vi "CyberSim.vi"() -> ()   [LabVIEW 2015]
doc: "Top-level VI to run one simulation of the iRobot and environment."
uses:
  CyberSim interface/Simulation Configuration.ctl
  autograder/feedbackMode.ctl
  shared/Kobuki Sensor Display.ctl
  <vilib>/Utility/miscctls.llb/LVRectTypeDef.ctl
  shared/Accelerometer.ctl
  <vilib>/Utility/miscctls.llb/LVPositionTypeDef.ctl
panel:
  out "size(s) 3":i32
  out "Display:Primary Workspace":T1
  out "Front Panel Window:Panel Bounds":T1
  in  "home camera":bool
  in  "stop":bool
  in  "start":bool
  in  "pause":bool
  in  "check grade":bool
  in  "exit":bool=TRUE
  out "Simulator Display":refnum<vi>(3d-picture)
  out "FullScreen":bool caption="--> Full Simulator Screens.\nPress \"ESC\" to exis full screen"
  in  "Change Sence":bool
  out "Sequence Number":i32
  out "Simulation Running":bool
  in  "Front Panel Tabs":T2(tab)=enum."Configuration"
  out "Statechart Diagram Display (supports LabVIEW Statecharts only)":picture
  out "Feedback":string
  in  "Simulation Configuration":T3={"maxTime"=inf, "enableVisualization"=TRUE, "Environment Definition"=path "Environment - Kobuki Hill Climb 1.xml", "Record Location"=path "Simulation Record.xml", "autograde?"=FALSE, "interactive?"=FALSE, "Feedback Mode"=enum."debug navigation", "Robot State Charts"=[path "../statechart/Simulation Statechart.vi"], "statechart"=path "../statechart/Simulation Statechart.vi"}
  in  "save configuration":bool
  in  "terminate at simulation end?":bool
  out "Simulation Time (s)":sgl=48.645 format="%7.3g"
  in  "play":bool
  out "?":T5={"Center Bump"=FALSE, "Left Wheel Drop"=FALSE, "Right Wheel Drop"=FALSE, "Left Bump"=FALSE, "Right Bump"=FALSE, "Left Cliff"=FALSE, "Center Cliff"=FALSE, "Right Cliff"=FALSE, "Net Dist (mm)"=3605, "Net Angle (deg)"=-38, "Left Cliff"=758, "Center Cliff"=770, "Right Cliff"=758, "  Left Wheel (mm/s)"=0, "Right Wheel (mm/s)"=0, "accelerometer"={"x axis (g)"=0.15724706555574047, "y axis (g)"=-0.0026101499423643627, "z axis (g)"=0.9842804420695141}} {"Right Wheel (mm/s)" scale=-500.0..500.0; "Left Wheel (mm/s)" scale=-500.0..500.0}
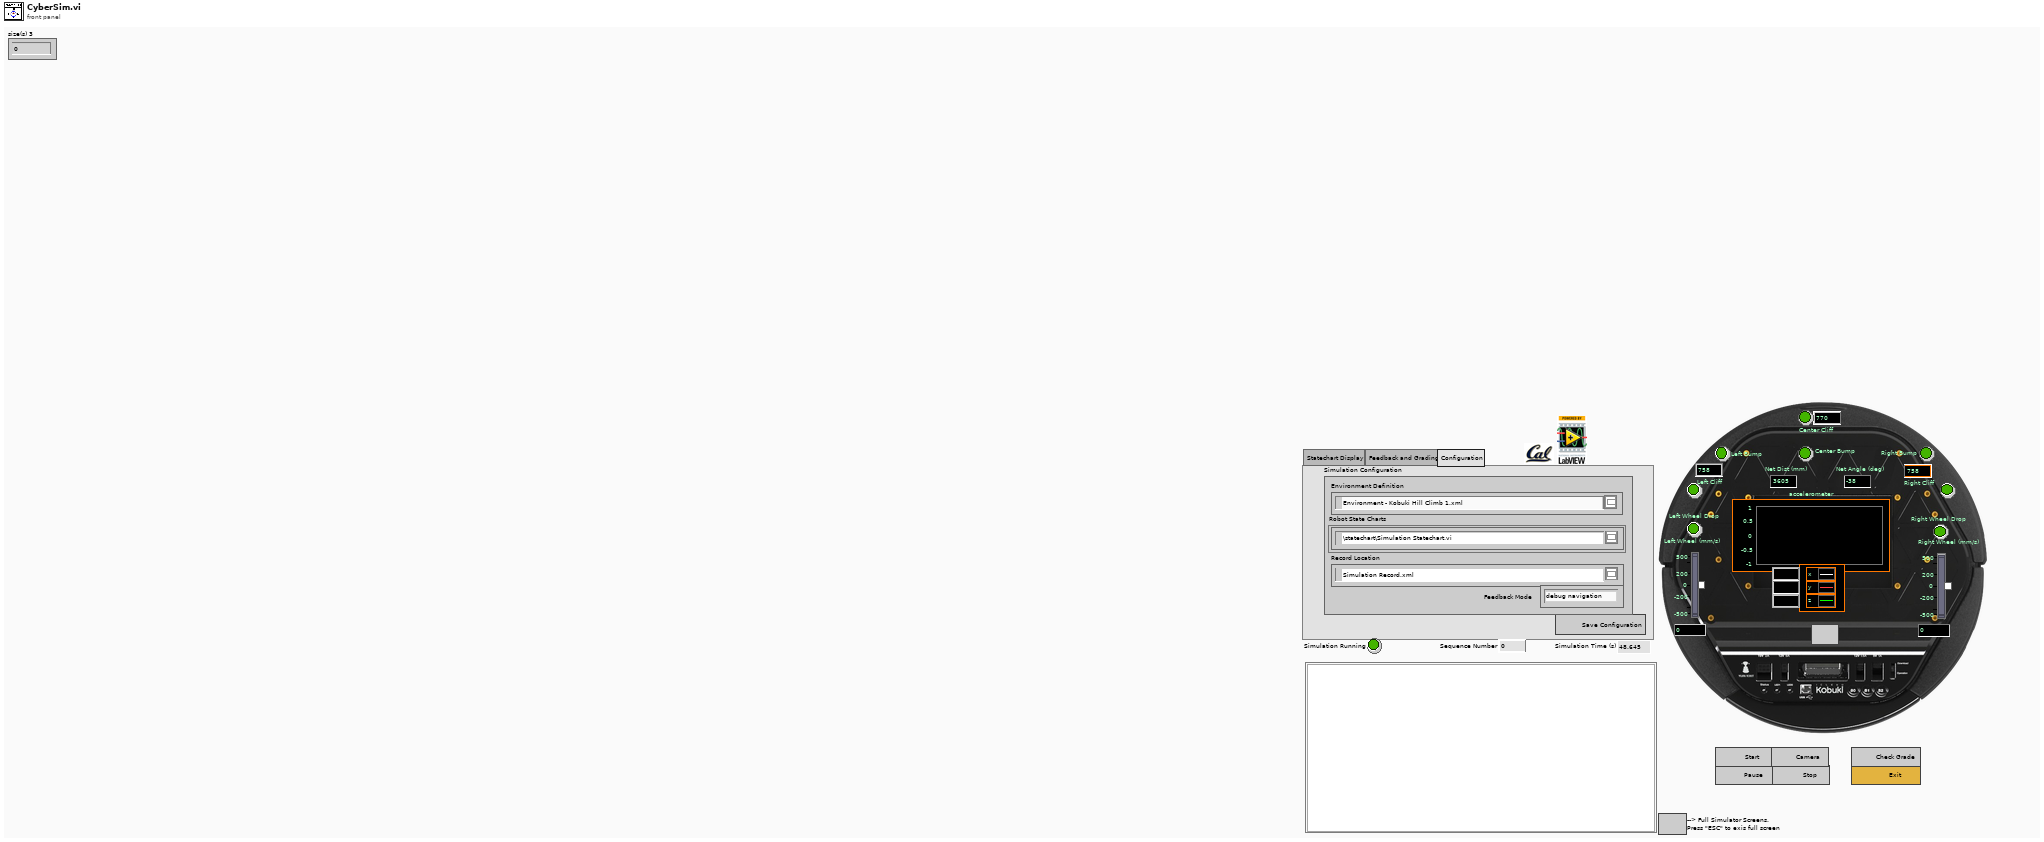
[diagram p1: front panel]
types:
  T1 = typedef "LVRectTypeDef.ctl" = cluster{"Left":i16, "Top":i16, "Right":i16, "Bottom":i16}
  T2 = enum32{"Statechart Display", "Feedback and Grading", "Configuration"}
  T3 = typedef "Simulation Configuration.ctl" = cluster{"maxTime":sgl, "enableVisualization":bool, "Environment Definition":path, "Record Location":path, "autograde?":bool, "interactive?":bool, "Feedback Mode":T4, "Robot State Charts":path[], "statechart":path}
  T4 = typedef "feedbackMode.ctl" = enum32{"debug navigation", "debug hill climb", "autograde navigation", "autograde hill climb"}
  T5 = typedef "Kobuki Sensor Display.ctl" = cluster{"Center Bump":bool, "Left Wheel Drop":bool, "Right Wheel Drop":bool, "Left Bump":bool, "Right Bump":bool, "Left Cliff":bool, "Center Cliff":bool, "Right Cliff":bool, "Net Dist (mm)":i32, "Net Angle (deg)":i32, "Left Cliff":u16, "Center Cliff":u16, "Right Cliff":u16, "  Left Wheel (mm/s)":i16, "Right Wheel (mm/s)":i16, "accelerometer":T6}
  T6 = typedef "Accelerometer.ctl" = cluster{"x axis (g)":dbl, "y axis (g)":dbl, "z axis (g)":dbl}
  T7 = typedef "LVPositionTypeDef.ctl" = cluster{"Left":i32, "Top":i32}
  T8 = enum16{"No Scaling", "Scale All Objects", "Scale Single Object"}
  T9 = enum16{"Always On", "Always Off", "Off While Running"}
  T10 = typedef "eventvkey.ctl" = enum16{"ASCII", "Enter", "Return", "Shift", "Ctrl", "Alt", "Cmd", "Opt", "Caps", "NumLock", "Clear", "Break", "Up", "Down", "Left", "Right", "Insert", "Delete", "Home", "End", "PageUp", "PageDown", "Escape", "Help", "Pause", "ScrollLock", "F1", "F2", "F3", "F4", "F5", "F6", "F7", "F8", "F9", "F10", "F11", "F12", "F13", "F14", "F15", "F16", "F17", "F18", "F19", "F20", "F21", "F22", "F23", "F24", "Play", "VolumeUp", "VolumeDown", "Mute", "Two Byte Char"}
  T11 = typedef "Simulator.ctl" = cluster{"configuration":T3, "Statechart\ndisplay":refnum<vi>, "first step?":bool, "Robots Simulation Statecharts":path[], "Robots":T12[]}
  T12 = typedef "RobotData.ctl" = cluster{"Bump Sensors":refnum<k20>[], "Distance Sensors":refnum<k20>[], "Accelerometer":refnum<k20>, "Wall Sensor":refnum<k20>, "Body":refnum<k20>, "RobotID":string, "RobotType":string, "Left Motor":refnum<class "DC Motor Controller.lvclass">, "Right Motor":refnum<class "DC Motor Controller.lvclass">}
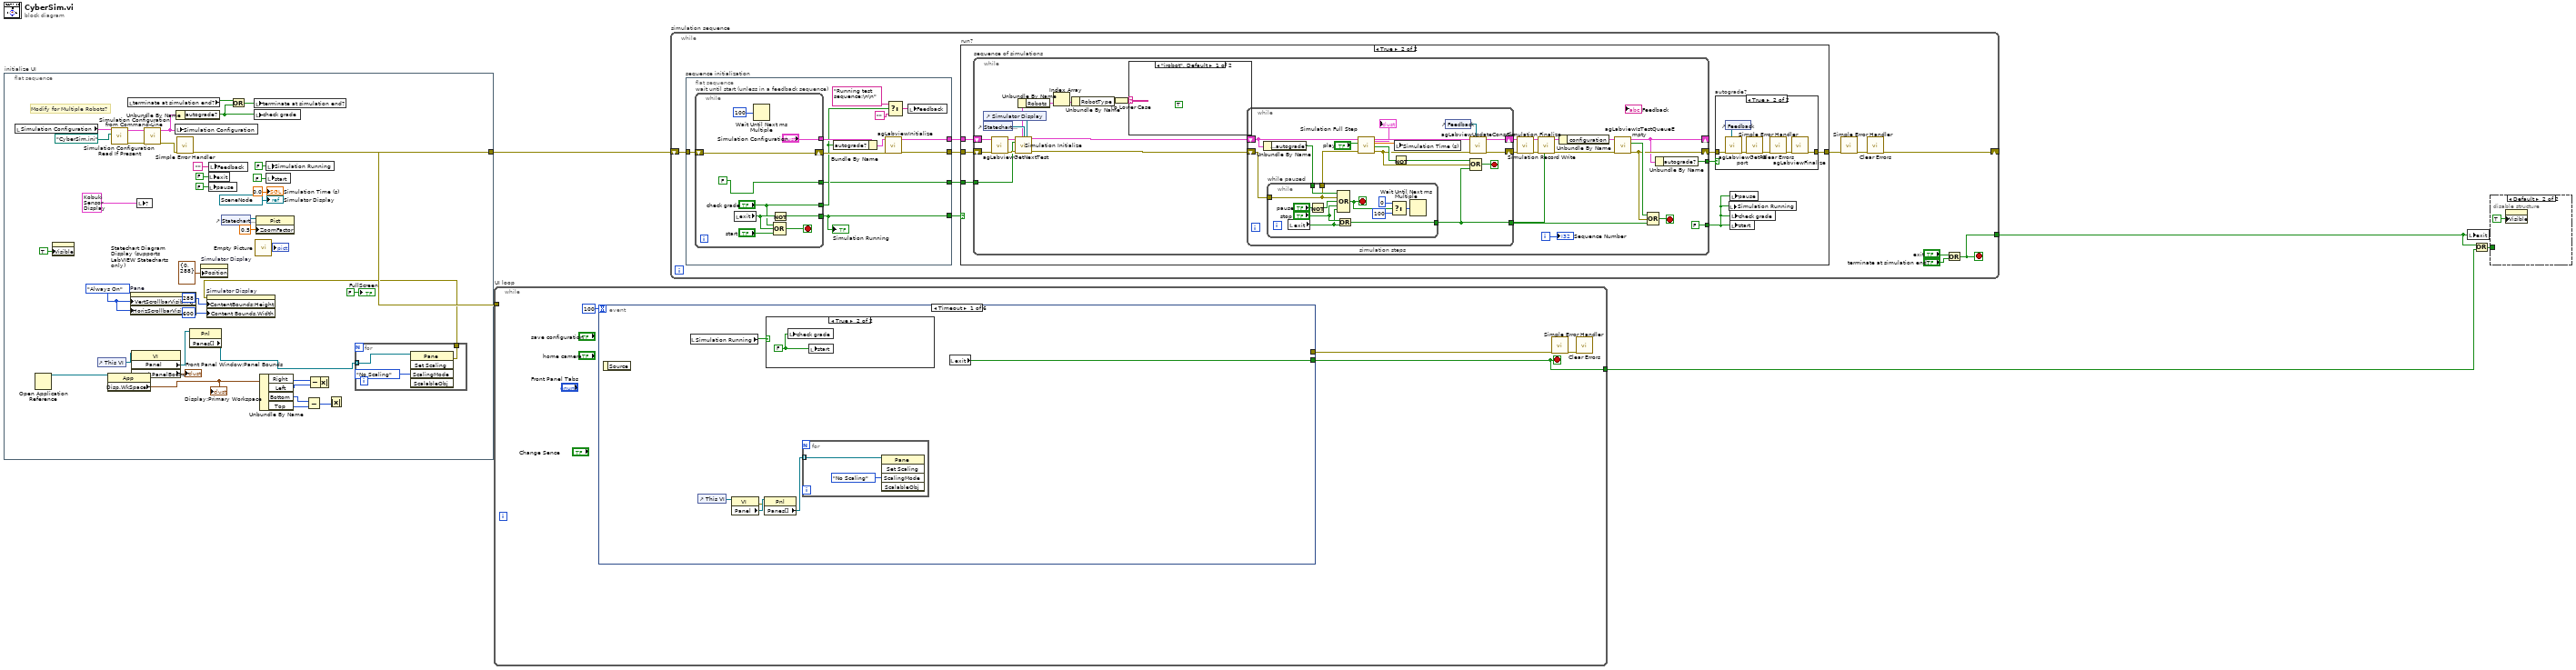
[diagram p0: block diagram]
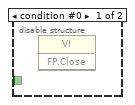
[diagram p2: hidden frame]
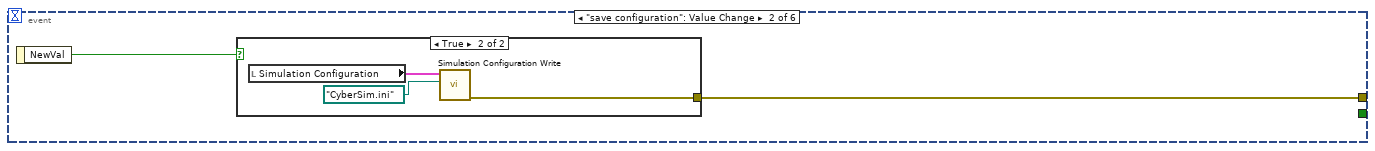
[diagram p4: hidden frame]
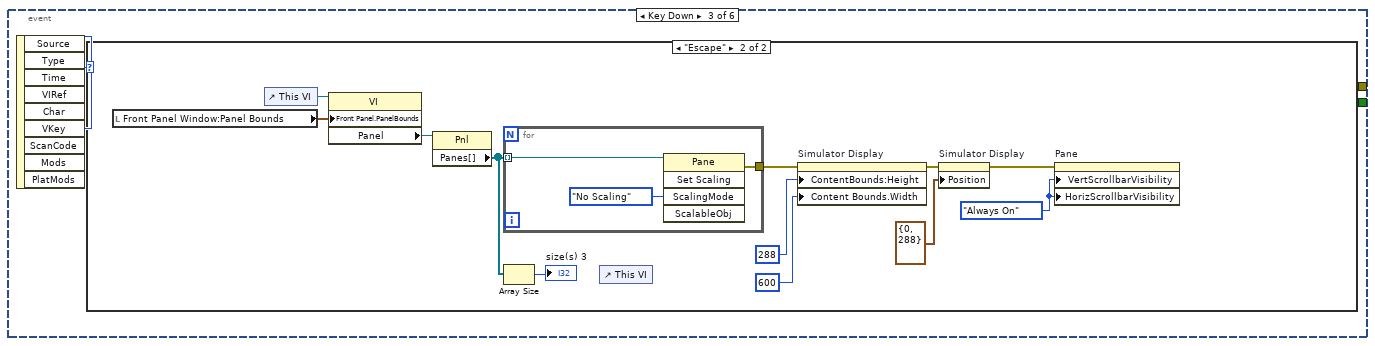
[diagram p6: hidden frame]
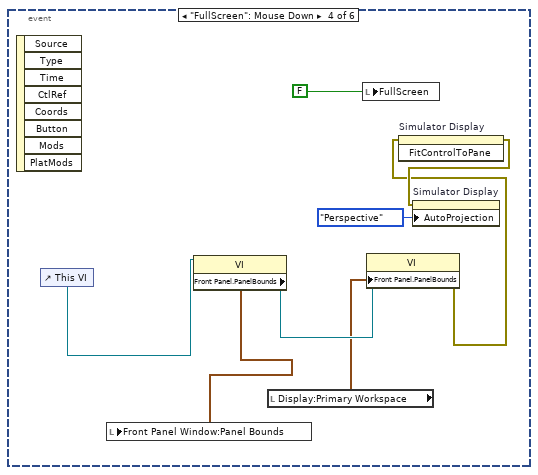
[diagram p8: hidden frame]
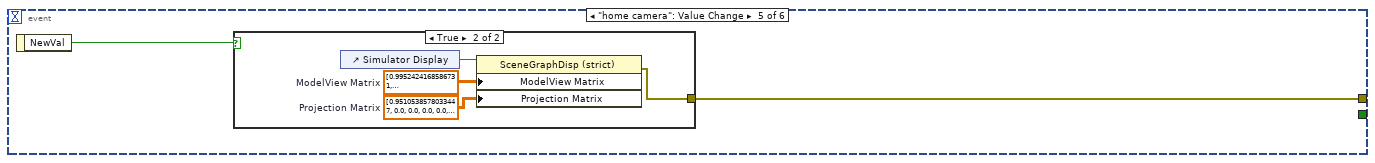
[diagram p9: hidden frame]
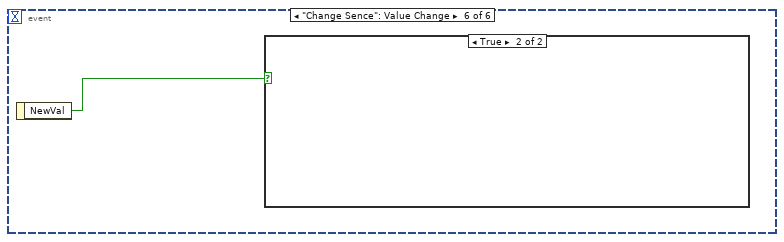
[diagram p11: hidden frame]
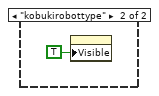
[diagram p15: hidden frame]
diagram:
  n1 = flat-sequence "initialize UI" {
    tunnel: [w41] -> w4
    frame #0 {
      w22 = T9."Always On" ("Horizontal Scrollbar Visibility")
      # "Modify for Multiple Robots?"
      n2 = local read "Simulation Configuration"() -> (w39:T3)
      n3 = Open Application Reference() -> (3:w14:refnum<vi>)  [unwired: 4 in, 1 out]
      n4 = property class="Clust (strict)"("Visible"=TRUE) -> ()  [unwired: 2 in, 2 out]
      n5 = control-ref of="This VI"() -> (w17:refnum<vi>)
      n6 = property class="App"(reference=w14) -> ("Disp.WkSpace"=w13:T1)  [unwired: 1 in, 2 out]
      "Display:Primary Workspace" <- w13
      n7 = call "Simulation Configuration Read If Present.vi"("configuration"=path "CyberSim.ini", "simulation configuration"=w39) -> ("error out"=w37:errorcluster, "simulation configuration"=w38:T3)  [unwired: 8 in]
      n8 = local read "terminate at simulation end?"() -> (w29:bool)
      n9 = property on="Pane" class="Pane"("VertScrollbarVisibility"=w22, "HorizScrollbarVisibility"=w22) -> ()  [unwired: 2 in, 2 out]
      n10 = property class="VI"(reference=w17) -> ("Panel"=w16:refnum<vi>, "Front Panel.PanelBounds"=→"Front Panel Window:Panel Bounds":T1)  [unwired: 1 in, 2 out]
      n11 = local write item#17(T5 {"Center Bump"=FALSE, "Left Wheel Drop"=FALSE, "Right Wheel Drop"=FALSE, "Left Bump"=FALSE, "Right Bump"=FALSE, "Left Cliff"=FALSE, "Center Cliff"=FALSE, "Right Cliff"=FALSE, "Net Dist (mm)"=0, "Net Angle (deg)"=0, "Left Cliff"=0, "Center Cliff"=0, "Right Cliff"=0, "  Left Wheel (mm/s)"=0, "Right Wheel (mm/s)"=0, "accelerometer"={"x axis (g)"=0.0, "y axis (g)"=0.0, "z axis (g)"=0.0}} ("Kobuki Sensors Display")) -> ()
      n12 = call "Simulation Configuration from Command-Line.vi"("error in"=w37, "simulation configuration in"=w38) -> ("error out"=w36:errorcluster, "simulation configuration out"=w34:T3)  [unwired: 8 in]
      n13 = local write "Simulation Configuration"(w34) -> ()
      n14 = Unbundle By Name(w34) -> ("autograde?"=w28:bool)
      n15 = call <vilib>:"Simple Error Handler.vi"("error in (no error)"=w36) -> ("error out"=w41:errorcluster)  [unwired: 4 in, 4 out]
      n16 = property class="Pnl"(reference=w16) -> ("Panes[]"=w15:refnum<vi>[])  [unwired: 1 in, 2 out]
      n17 = property on="Simulator Display" class="SceneGraphDisp (strict)"("Position"=T7 {"Left"=0, "Top"=288}) -> ()  [unwired: 2 in, 2 out]
      n18 = local write "exit"(FALSE ("exit")) -> ()
      n19 = local write "pause"(FALSE ("pause")) -> ()
      n20 = local write "Feedback"("") -> ()
      n21 = control-ref of="Statechart Diagram Display (supports LabVIEW Statecharts only)"() -> (w26:refnum<vi>)
      n22 = Or(x=w29, y=w28) -> (x .or. y?=w30:bool)
      n23 = local write "terminate at simulation end?"(w30) -> ()
      n24 = local write "check grade"(w28) -> ()
      n25 = call "Empty Picture"() -> ("empty picture"=→"Statechart Diagram Display (supports LabVIEW Statecharts only)":picture)
      n26 = property class="Pict"(reference=w26, "ZoomFactor"=sgl 0.5 ("Zoom Factor")) -> ()  [unwired: 1 in, 2 out]
      n27 = Unbundle By Name(w13) -> ("Right"=w12:i16, "Left"=w11:i16, "Bottom"=w9:i16, "Top"=w8:i16)
      n28 = local write "Simulation Running"(FALSE ("simulation running")) -> ()
      n29 = local write "start"(FALSE ("start")) -> ()
      n30 = Subtract(x=w9, y=w8) -> (x-y=w7:i16)
      n31 = Subtract(x=w12, y=w11) -> (x-y=w10:i16)
      n32 = Absolute Value(x=w10) -> ()  [unwired: 1 out]
      n33 = Absolute Value(x=w7) -> ()  [unwired: 1 out]
      n34 = for {
        tunnel: w15 -> [w47] mode=indexing
        tunnel: [w45] -> w5
        n35 = invoke class="Pane" method="Set Scaling"(reference=w47, "ScalingMode"=T8."No Scaling" ("Scaling Mode")) -> (error out=w45:errorcluster)  [unwired: 3 in, 4 out]
      }
      n36 = property on="Simulator Display" class="SceneGraphDisp (strict)"(error in=w5, "ContentBounds:Height"=u32 288 ("Content Bounds:Height"), "Content Bounds.Width"=u32 600 ("Content Bounds:Width")) -> ()  [unwired: 1 in, 2 out]
      "Simulation Time (s)" <- sgl 0.0 ("simulated time (s)")
      "Simulator Display" <- refnum<vi> refnum ("3D Picture")
      "FullScreen" <- FALSE
    }
  }
  n37 = while "UI loop" {
    tunnel: [w49] -> w2
    tunnel: w4 -> [_]
    stop <- w49 stop-if-true
    n38 = event shown="[0] Timeout" {
      selector: _ -> [_ _ _ _ _ _]
      dyn-events: _ -> [_ _ _ _ _ _]
      timeout: 100 -> [_ _ _ _ _ _]
      tunnel: [_ w61 _ _ w90 _] -> w50
      tunnel: [w57 _ _ _ _ _] -> w49
      event Timeout {
        n39 = event-data() -> ()  [unwired: 1 in, 1 out]
        n40 = local read "Simulation Running"() -> (w56:bool)
        n41 = control-ref of="This VI"() -> (w55:refnum<vi>)
        n42 = property class="VI"(reference=w55) -> (error out=w52:errorcluster, "Panel"=w53:refnum<vi>)  [unwired: 1 in, 1 out]
        n43 = property class="Pnl"(reference=w53, error in=w52) -> ("Panes[]"=w54:refnum<vi>[])  [unwired: 2 out]
        n44 = case shown="True" w56 {
          frame False {
          }
          frame True {
            w60 = FALSE ("AutoGrade")
            n45 = local write "check grade"(w60) -> ()
            n46 = local write "start"(w60) -> ()
          }
        }
        n47 = for {
          tunnel: w54 -> [w59] mode=indexing
          n48 = invoke class="Pane" method="Set Scaling"(reference=w59, "ScalingMode"=T8."No Scaling" ("Scaling Mode")) -> ()  [unwired: 3 in, 5 out]
        }
        n49 = local read "exit"() -> (w57:bool)
      }
      event "save configuration": Value Change {
        n50 = event-data() -> ("NewVal"=w62:bool)  [unwired: 1 in]
        n51 = case shown="True" w62 {
          tunnel: [_ w64] -> w61
          frame False {
          }
          frame True {
            n52 = local read "Simulation Configuration"() -> (w65:T3)
            n53 = call "Simulation Configuration Write.vi"("configuration"=path "CyberSim.ini", "simulation configuration"=w65) -> ("error out"=w64:errorcluster)  [unwired: 9 in]
          }
        }
      }
      event Key Down {
        n54 = event-data() -> ("VKey"=w66:T10)  [unwired: 1 in, 8 out]
        n55 = case shown="\"Escape\"" w66 {
          frame "ASCII", Default {
          }
          frame "Escape" {
            w78 = T9."Always On" ("Horizontal Scrollbar Visibility")
            n56 = local read "Front Panel Window:Panel Bounds"() -> (w71:T1)
            n57 = control-ref of="This VI"() -> (w74:refnum<vi>)
            n58 = property class="VI"(reference=w74, "Front Panel.PanelBounds"=w71) -> ("Panel"=w68:refnum<vi>)  [unwired: 1 in, 2 out]
            n59 = property class="Pnl"(reference=w68) -> ("Panes[]"=w69:refnum<vi>[])  [unwired: 1 in, 2 out]
            n60 = for {
              tunnel: w69 -> [w81] mode=indexing
              tunnel: [w79] -> w67
              n61 = invoke class="Pane" method="Set Scaling"(reference=w81, "ScalingMode"=T8."No Scaling" ("Scaling Mode")) -> (error out=w79:errorcluster)  [unwired: 3 in, 4 out]
            }
            n62 = Array Size(array=w69) -> (size(s)=→"size(s) 3":i32)
            n63 = control-ref of="This VI"() -> ()  [unwired: 1 out]
            n64 = property on="Simulator Display" class="SceneGraphDisp (strict)"(error in=w67, "ContentBounds:Height"=u32 288 ("Content Bounds:Height"), "Content Bounds.Width"=u32 600 ("Content Bounds:Width")) -> (error out=w73:errorcluster)  [unwired: 1 in, 1 out]
            n65 = property on="Simulator Display" class="SceneGraphDisp (strict)"(error in=w73, "Position"=T7 {"Left"=0, "Top"=288}) -> (error out=w72:errorcluster)  [unwired: 1 in, 1 out]
            n66 = property on="Pane" class="Pane"(error in=w72, "VertScrollbarVisibility"=w78, "HorizScrollbarVisibility"=w78) -> ()  [unwired: 1 in, 2 out]
          }
        }
      }
      event "FullScreen": Mouse Down {
        n67 = event-data() -> ()  [unwired: 1 in, 8 out]
        n68 = control-ref of="This VI"() -> (w86:refnum<vi>)
        n69 = property class="VI"(reference=w86) -> (reference out=w85:refnum<vi>, "Front Panel.PanelBounds"=w83:T1)  [unwired: 1 in, 1 out]
        n70 = local write "Front Panel Window:Panel Bounds"(w83) -> ()
        n71 = local read "Display:Primary Workspace"() -> (w82:T1)
        n72 = local write "FullScreen"(FALSE ("Maximize Simulator Screens")) -> ()
        n73 = property class="VI"(reference=w85, "Front Panel.PanelBounds"=w82) -> (error out=w84:errorcluster)  [unwired: 1 in, 1 out]
        n74 = invoke on="Simulator Display" class="SceneGraphDisp (strict)" method="FitControlToPane"(error in=w84) -> (error out=w87:errorcluster)  [unwired: 2 in, 2 out]
        n75 = property on="Simulator Display" class="SceneGraphDisp (strict)"(error in=w87, "AutoProjection"=enum16{"None", "Perspective", "Orthographic"}."Perspective" ("Automatic Projection Mode")) -> ()  [unwired: 1 in, 2 out]
      }
      event "home camera": Value Change {
        n76 = event-data() -> ("NewVal"=w91:bool)  [unwired: 1 in]
        n77 = case shown="True" w91 {
          tunnel: [_ w92] -> w90
          frame False {
          }
          frame True {
            w93 = sgl[][] [[0.95105386, 0.0, 0.0, 0.0], [0.0, 2.4142137, 0.0, 0.0], [0.0, 0.0, -1.0002, -0.020002], [0.0, 0.0, -1.0, 0.0]]  # Projection Matrix
            w94 = sgl[][] [[0.9952424, -0.09162651, 0.033122927, -2.4552457], [0.010721975, 0.44090375, 0.8974903, -1.0543748], [-0.09683793, -0.8928653, 0.43978852, -0.9396557], [0.0, 0.0, 0.0, 1.0]]  # ModelView Matrix
            n78 = control-ref of="Simulator Display"() -> (w95:refnum<vi>)
            n79 = property class="SceneGraphDisp (strict)"(reference=w95, "ModelView Matrix"=w94, "Projection Matrix"=w93) -> (error out=w92:errorcluster)  [unwired: 1 in, 1 out]
          }
        }
      }
      event "Change Sence": Value Change {
        n80 = event-data() -> ("NewVal"=w96:bool)  [unwired: 1 in]
        n81 = case shown="True" w96 {
          frame False {
          }
          frame True {
          }
        }
      }
    }
    n82 = call <vilib>:"Simple Error Handler.vi"("error in (no error)"=w50) -> ("error out"=w48:errorcluster)  [unwired: 4 in, 4 out]
    n83 = call <vilib>:"Clear Errors.vi"("error in (no error)"=w48) -> ()  [unwired: 5 in, 2 out]
  }
  n84 = while "simulation sequence" {
    tunnel: [w104] -> w3
    shift-right: [w102] -> _
    shift-left: w4 -> [w98]
    stop <- w104 stop-if-true
    n85 = flat-sequence "sequence initialization" {
      tunnel: [w188] -> w103
      tunnel: [w189] -> w101
      tunnel: [w184] -> w100
      tunnel: w98 -> [w187]
      tunnel: [w179] -> w97
      frame #0 {
        n86 = while "wait until start (unless in a feedback sequence)" {
          shift-right: [w195] -> w186
          shift-left: w187 -> [w195]
          tunnel: ["check grade"] -> w183
          tunnel: ["Simulation Configuration"] -> w185
          tunnel: [w192] -> w184
          tunnel: [FALSE ("start 2")] -> w179
          stop <- w199 stop-if-true
          n87 = local read "exit"() -> (w198:bool)
          n88 = Wait Until Next ms Multiple(millisecond multiple=u32 100) -> ()  [unwired: 1 out]
          n89 = Not(x=w198) -> (.not. x?=w192:bool)
          n90 = Compound Arithmetic op=OR("check grade", w198, "start") -> (w199:bool)
        }
        "Simulation Running" <- w184
        n91 = Bundle By Name(cluster=w185, "autograde?"=w183) -> (w190:T3)
        n92 = call "agLabviewInitialize.vi"("Error In"=w186, "simulation configuration"=w190) -> ("Error Out"=w189:errorcluster, "simulation configuration"=w188:T3)  [unwired: 8 in]
        n93 = Select(t="Running test sequence:\n\n", s=w183, f="") -> (s? t:f=w181:string)
        n94 = local write "Feedback"(w181) -> ()
      }
    }
    n95 = case "run?" shown="True" w100 {
      tunnel: w103 -> [_ w115]
      tunnel: w101 -> [w108 w114]
      tunnel: [w108 w111] -> w99
      tunnel: w97 -> [_ w109]
      frame False {
      }
      frame True {
        n96 = while "sequence of simulations" {
          shift-right: [w139] -> w112
          shift-left: w114 -> [w134]
          shift-right: [w129] -> _
          shift-left: w115 -> [w133]
          tunnel: [w138] -> w113
          tunnel: [FALSE] -> w110
          tunnel: w109 -> [w128]
          i -> [w150]
          stop <- w149 stop-if-true
          n97 = control-ref of="Simulator Display"() -> (w145:refnum<vi>)
          n98 = control-ref of="Statechart Diagram Display (supports LabVIEW Statecharts only)"() -> (w147:refnum<vi>)
          n99 = call "agLabviewGetNextTest.vi"("Error In"=w134, "simulation configuration"=w133) -> ("Error Out"=w135:errorcluster, "simulation configuration"=w136:T3)  [unwired: 8 in]
          n100 = call "Simulation Initialize.vi"("simulation configuration"=w136, "Statechart display"=w147, "Simulator display"=w145, "Real Time"=w128, "Error In"=w135) -> ("simulator"=w123:T11, "Error Out"=w148:errorcluster)  [unwired: 9 in]
          n101 = Unbundle By Name(w123) -> ("Robots"=w127:T12[])
          n102 = Index Array(array=w127) -> (element=w126:T12)  [unwired: 1 in]
          n103 = Unbundle By Name(w126) -> ("RobotType"=w125:string)
          n104 = To Lower Case(string=w125) -> (all lower case string=w124:string)
          n105 = case shown="\"irobot\", Default" w124 {
            frame "irobot", Default {
              (unwired) TRUE ("Visible")
            }
            frame "kobukirobottype" {
              n106 = property class="Clust (strict)"("Visible"=TRUE) -> ()  [unwired: 2 in, 2 out]
            }
          }
          n107 = while "simulation steps" {
            shift-right: [w155] -> w144
            shift-left: w123 -> [w161]
            shift-right: [w154] -> w146
            shift-left: w148 -> [w159]
            tunnel: [w162] -> w140
            stop <- w166 stop-if-true
            n108 = Unbundle By Name(w161) -> ("configuration.autograde?"=w160:bool)
            n109 = while "while paused" {
              tunnel: [w174] -> w162
              tunnel: w159 -> [w168]
              tunnel: w160 -> [w169]
              tunnel: [w168] -> w158
              stop <- w170 stop-if-true
              n110 = local read "exit"() -> (w175:bool)
              n111 = Not(x="pause") -> (.not. x?=w177:bool)
              n112 = Or(x="stop", y=w175) -> (x .or. y?=w174:bool)
              n113 = Compound Arithmetic op=OR(w169, w168, w177, "stop", w175) -> (w170:bool)
              n114 = Select(t=u32 0 ("millisecond multiple"), s=w170, f=u32 100 ("millisecond multiple")) -> (s? t:f=w173:u32)
              n115 = Wait Until Next ms Multiple(millisecond multiple=w173) -> ()  [unwired: 1 out]
            }
            n116 = call "Simulation Full Step.vi"("Error In"=w158, "Play Button (false)"="play", "simulator"=w161) -> ("Error Out"=w157:errorcluster, "continue to next step?"=w167:bool, "simulated time (s)"=w164:sgl, "simulator"=w156:T11, "Kobuki Sensors Display"=→"?":T5)  [unwired: 4 in]
            n117 = Not(x=w167) -> (.not. x?=w163:bool)
            n118 = local write "Simulation Time (s)"(w164) -> ()
            n119 = control-ref of="Feedback"() -> (w153:refnum<vi>)
            n120 = call "agLabviewUpdateConsole.vi"("console"=w153, "Error In"=w157, "simulator"=w156) -> ("Error Out"=w154:errorcluster, "simulator"=w155:T11)  [unwired: 7 in]
            n121 = Compound Arithmetic op=OR(w163, w157, w162) -> (w166:bool)
          }
          n122 = call "Simulation Record Write.vi"("Error In"=w146, "simulator"=w144) -> ("Error Out"=w142:errorcluster, "simulator"=w143:T11)  [unwired: 8 in]
          n123 = call "Simulation Finalize.vi"("terminated by user?"=w140, "error in (no error)"=w142, "simulator"=w143) -> ("error out"=w131:errorcluster, "simulator"=w132:T11)  [unwired: 7 in]
          n124 = Unbundle By Name(w132) -> ("configuration"=w130:T3)
          n125 = call "agLabviewIsTestQueueEmpty.vi"("Error In"=w131, "simulation configuration"=w130) -> ("Error Out"=w139:errorcluster, "Empty?"=w141:bool, "simulation configuration"=w129:T3)  [unwired: 7 in]
          n126 = Compound Arithmetic op=OR(w141, w139, w140) -> (w149:bool)
          n127 = Unbundle By Name(w129) -> ("autograde?"=w138:bool)
          "Sequence Number" <- w150
        }
        n128 = case "autograde?" shown="True" w113 {
          tunnel: [w116 w122] -> w111
          tunnel: w112 -> [w116 w121]
          frame False {
          }
          frame True {
            n129 = control-ref of="Feedback"() -> (w120:refnum<vi>)
            n130 = call "agLabviewGetReport.vi"("console"=w120, "Error In"=w121) -> ("Error Out"=w118:errorcluster)  [unwired: 9 in]
            n131 = call <vilib>:"Simple Error Handler.vi"("error in (no error)"=w118) -> ("error out"=w119:errorcluster)  [unwired: 4 in, 4 out]
            n132 = call <vilib>:"Clear Errors.vi"("error in (no error)"=w119) -> ("error out"=w117:errorcluster)  [unwired: 5 in, 1 out]
            n133 = call "agLabviewFinalize.vi"("Error In"=w117) -> ("Error Out"=w122:errorcluster)  [unwired: 10 in]
          }
        }
        n134 = local write "Simulation Running"(w110) -> ()
        n135 = local write "pause"(w110) -> ()
        n136 = local write "check grade"(w110) -> ()
        n137 = local write "start"(w110) -> ()
      }
    }
    n138 = call <vilib>:"Simple Error Handler.vi"("error in (no error)"=w99) -> ("error out"=w107:errorcluster)  [unwired: 4 in, 4 out]
    n139 = call <vilib>:"Clear Errors.vi"("error in (no error)"=w107) -> ("error out"=w102:errorcluster)  [unwired: 5 in, 1 out]
    n140 = Or(x="exit", y="terminate at simulation end?") -> (x .or. y?=w104:bool)
  }
  n141 = local write "exit"(w3) -> ()
  n142 = Or(x=w3, y=w2) -> (x .or. y?=w1:bool)
  n143 = disable-structure shown="Default" {
    disable-tunnel: w1 -> [_ _]
    frame condition #0 {
      n144 = invoke class="VI" method="FP.Close"() -> ()  [unwired: 3 in, 3 out]
    }
    frame condition #1 (active) {
      n145 = property class="Clust (strict)"("Visible"=TRUE) -> ()  [unwired: 2 in, 2 out]
    }
  }
